vi "__Cloud List Menu Handler.vi"(7 "FileManager Data":T1, 8 "error in (no error)":errorcluster, 11 "Menuitem Tag":string) -> (0 "error out":errorcluster)   [LabVIEW 2011]
doc: "Handles the cloud list right-click menu."
uses:
  __File manager Data type.ctl
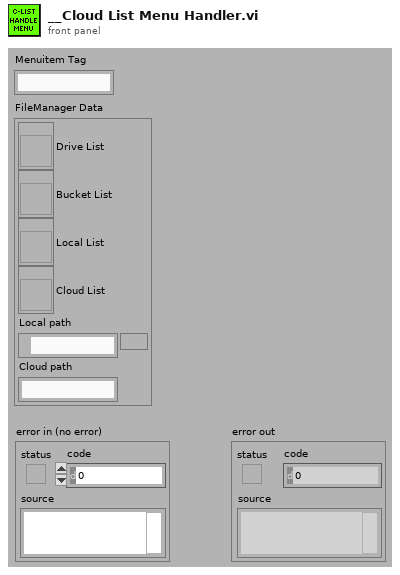
[diagram p1: front panel]
types:
  T1 = typedef "__File manager Data type.ctl" = cluster{"Drive List":refnum<vi>, "Bucket List":refnum<vi>, "Local List":refnum<vi>, "Cloud List":refnum<vi>, "Local path":path, "Cloud path":string}
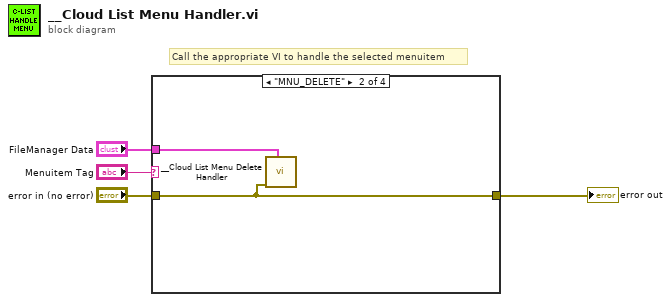
[diagram p0: block diagram]
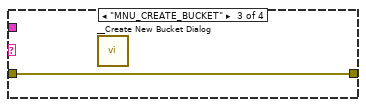
[diagram p3: hidden frame]
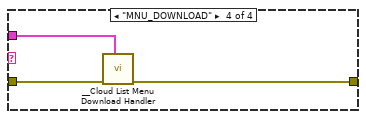
[diagram p4: hidden frame]
diagram:
  # "Call the appropriate VI to handle the selected menuitem"
  n1 = case shown="\"MNU_DELETE\"" "Menuitem Tag" {
    tunnel: "error in (no error)" -> [w5 w7 w8 w11]
    tunnel: [w5 w7 w8 w10] -> w2
    tunnel: "FileManager Data" -> [_ w6 _ w9]
    frame Default {
    }
    frame "MNU_DELETE" {
      n2 = call "__Cloud List Menu Delete Handler.vi"("FileManager Data"=w6, "error in (no error)"=w7) -> ()  [unwired: 9 in, 1 out]
    }
    frame "MNU_CREATE_BUCKET" {
      n3 = call "__Create New Bucket Dialog.vi"() -> ()  [unwired: 12 in]
    }
    frame "MNU_DOWNLOAD" {
      n4 = call "__Cloud List Menu Download Handler.vi"("FileManager Data"=w9, "error in (no error)"=w11) -> ("error out"=w10:errorcluster)  [unwired: 9 in]
    }
  }
  "error out" <- w2
